vi "SpreadsheetFGV2_Improvements.vi"(0 "Student ID":i32, 1 "FGV Control":T1, 11 "Error In":errorcluster) -> (3 "Time Stamp Out":timestamp, 4 "Message":string, 6 "Names":string[](array[string]), 8 "Output 2D Data":string[][](array[string]), 10 "Checked In?":bool, 12 "Cat Points":i32, 14 "Elapsed Time":dbl, 15 "Error Out":errorcluster)   [LabVIEW 2013]
uses:
  Controls/CSVFGVStates.ctl
  Controls/SpreadsheetColumns.ctl
  <vilib>/Utility/file.llb/Write To Spreadsheet File (string).vi
  <vilib>/Utility/file.llb/Read From Spreadsheet File (string).vi
panel:
  out "Checked In":string
  out "all rows":string[][](array[string])
  in  "Replacement":string
  in  "Student Names":i32(listbox)
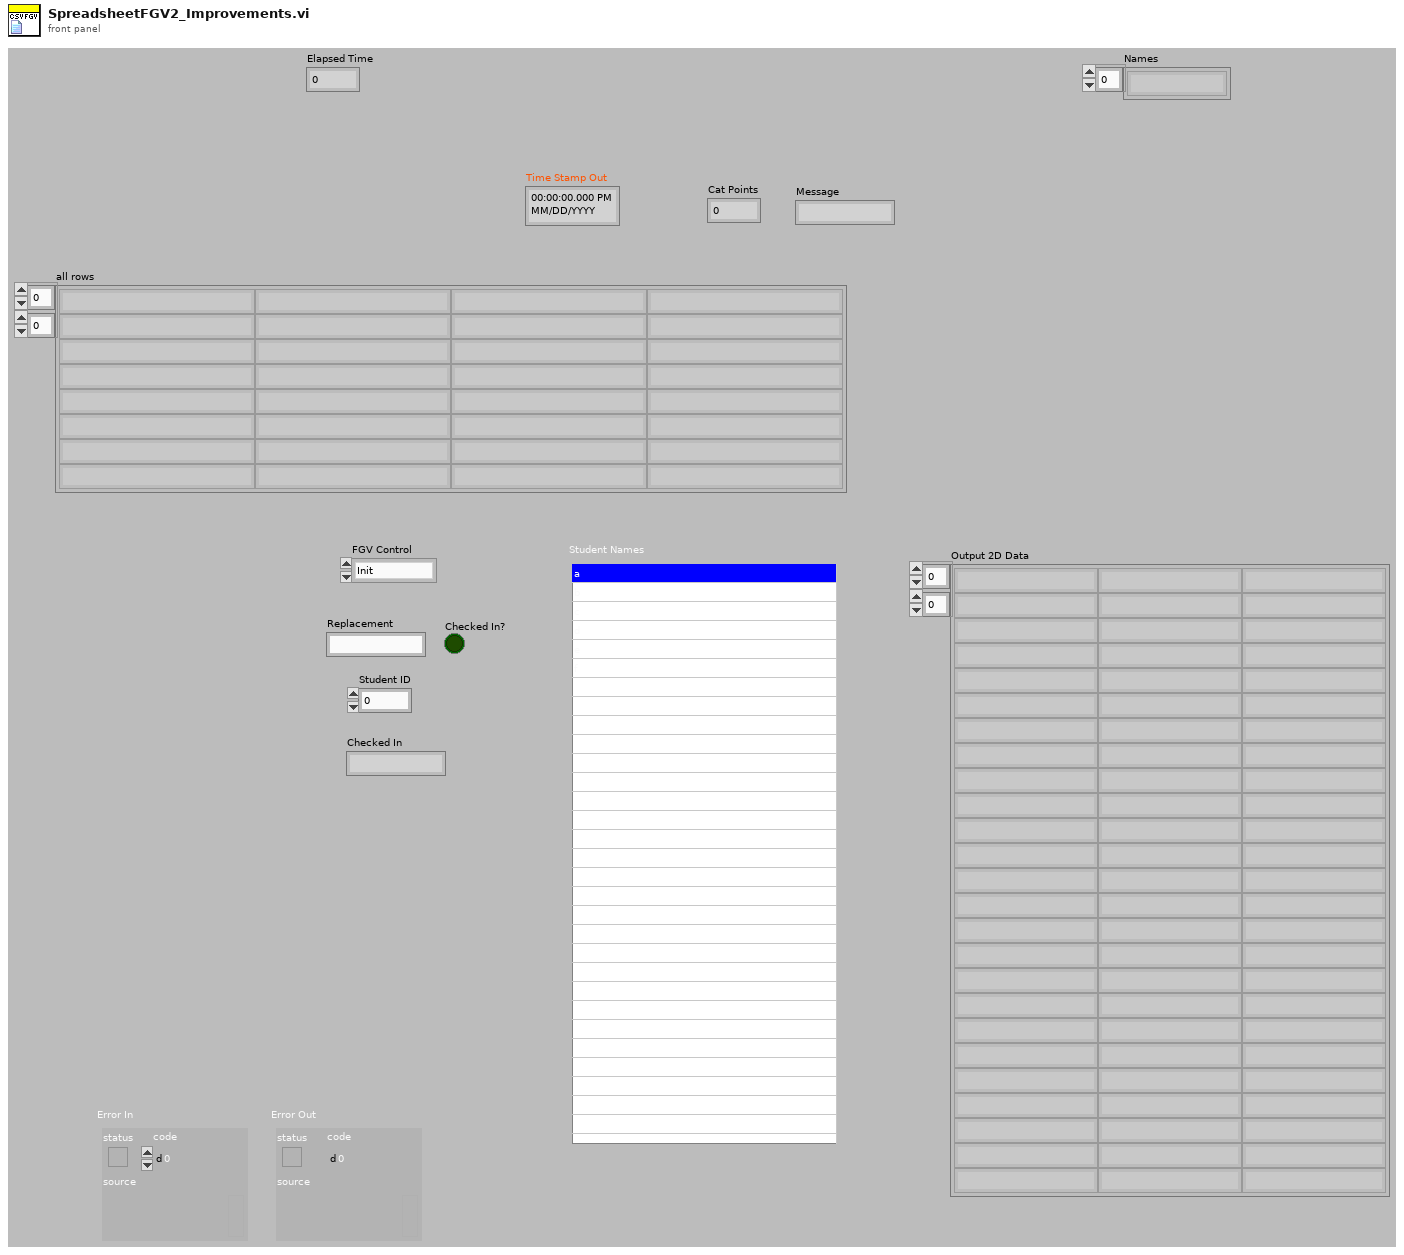
[diagram p1: front panel]
types:
  T1 = typedef "CSVFGVStates.ctl" = enum16{"Init", "Sort", "Check In", "Check Out", "Check Status", "Read CSV", "Close Out"}
  T2 = typedef "SpreadsheetColumns.ctl" = enum16{"Email", "CheckIn", "CheckOut", "Flag", "Hours", "Minutes", "Seconds", "Total Seconds", "Cat Points"}
  T3 = cluster{"Flag":T2, "Check In":T2, "Hours":T2, "Minutes":T2, "Seconds":T2, "Check Out":T2, "Email":T2, "Total Seconds":T2}
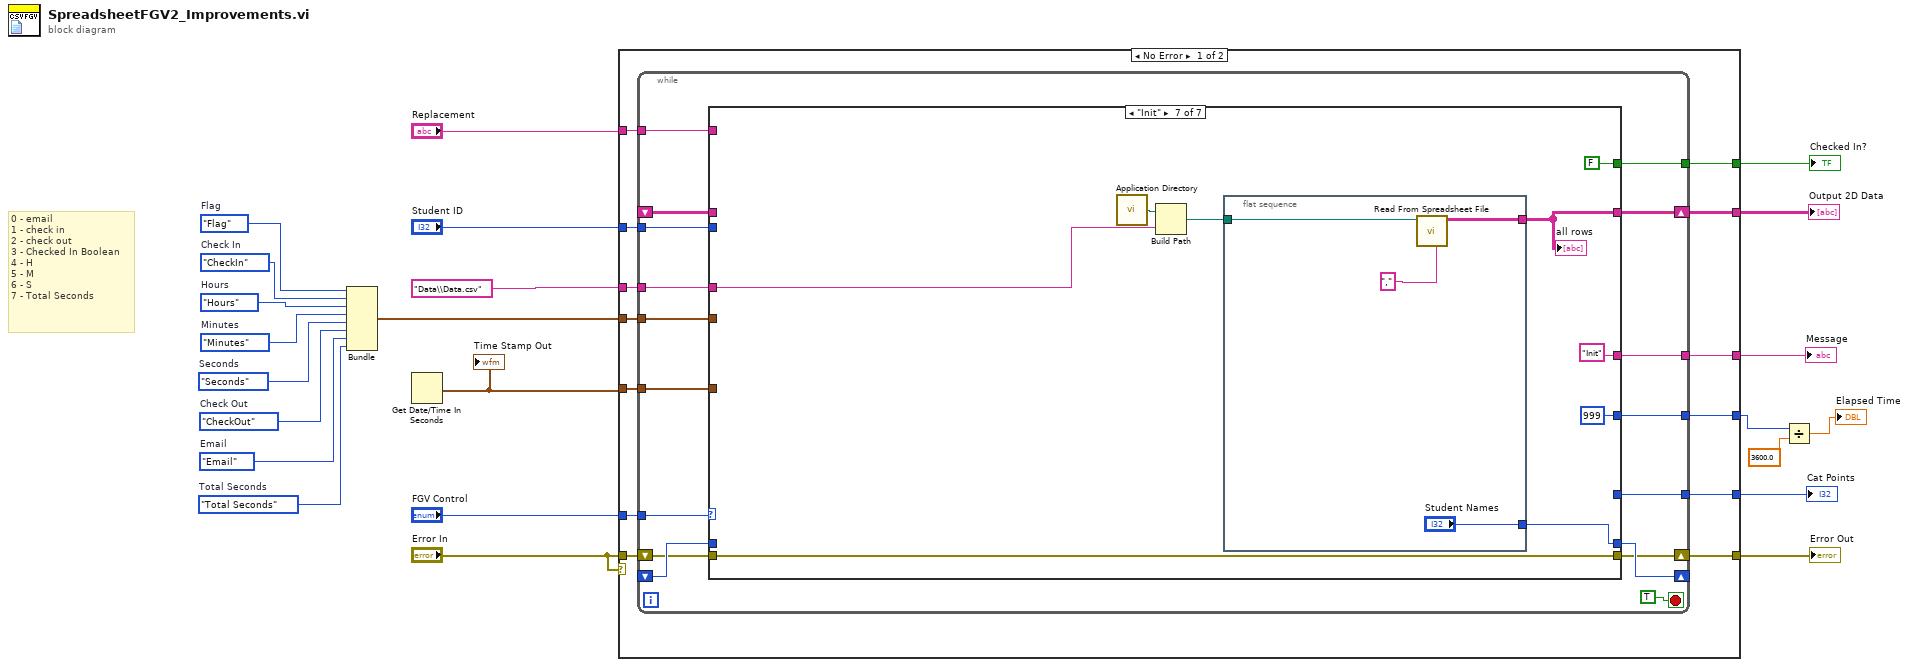
[diagram p0: block diagram]
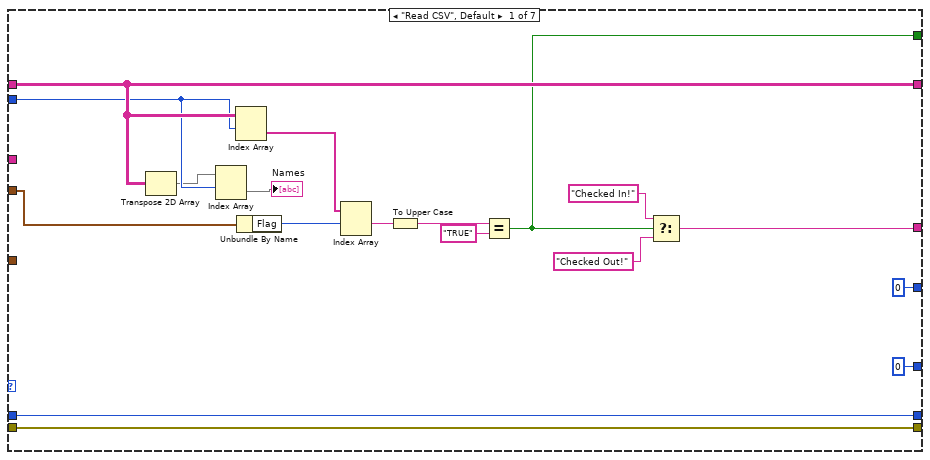
[diagram p2: hidden frame]
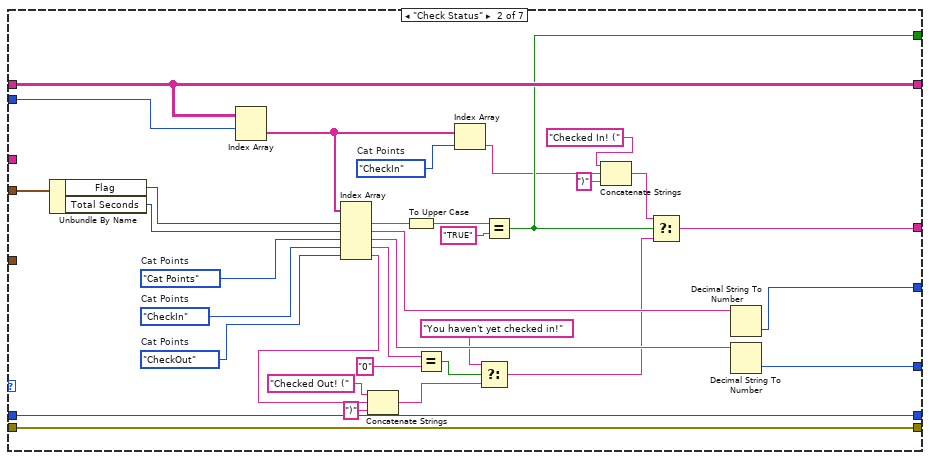
[diagram p3: hidden frame]
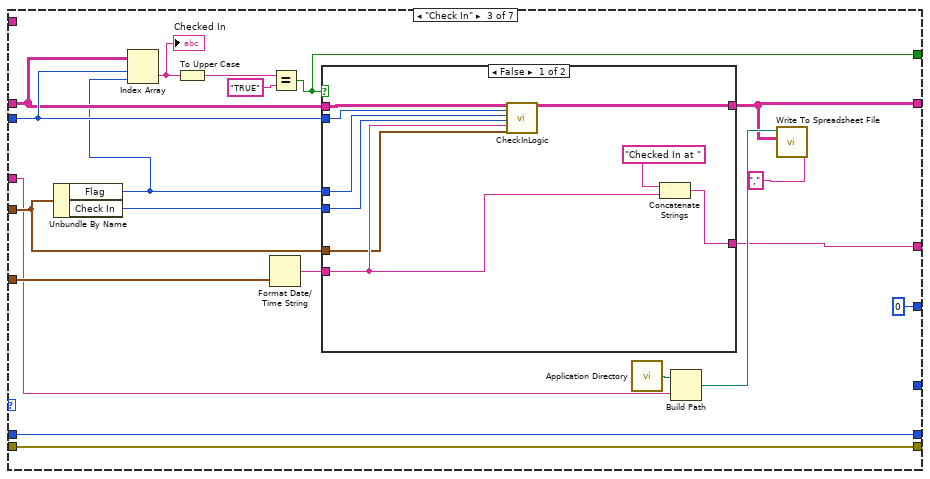
[diagram p4: hidden frame]
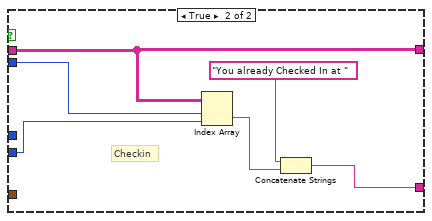
[diagram p5: hidden frame]
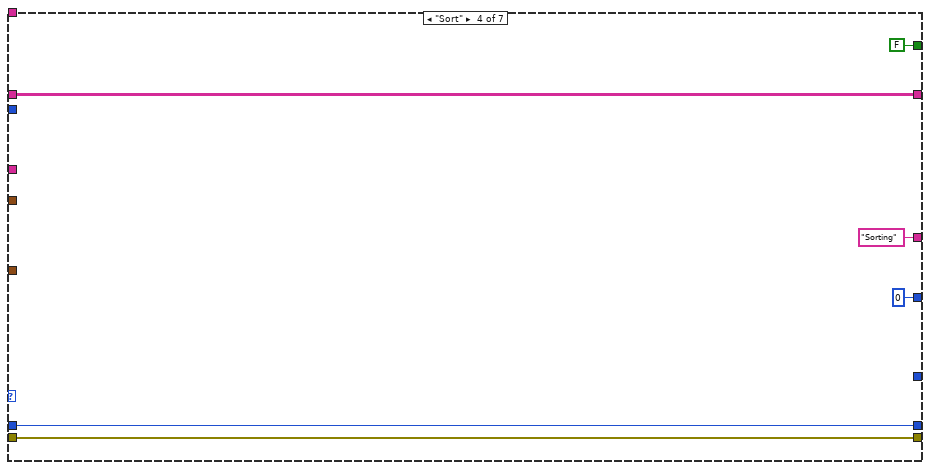
[diagram p6: hidden frame]
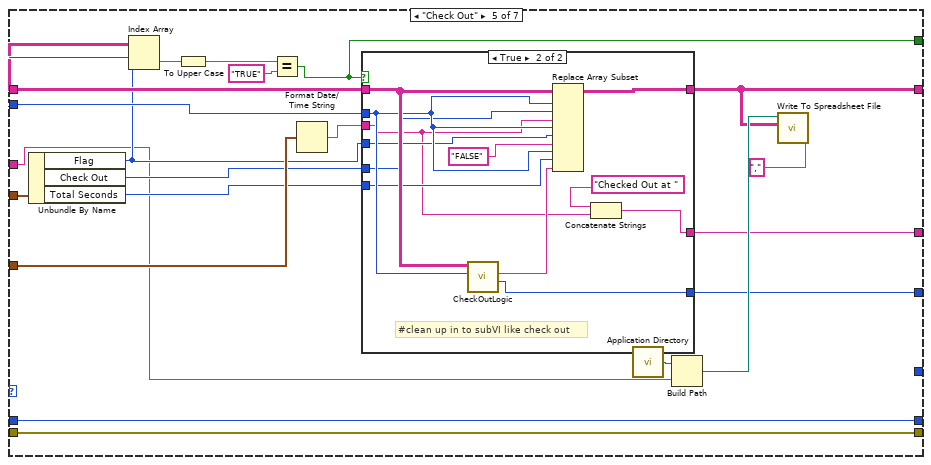
[diagram p7: hidden frame]
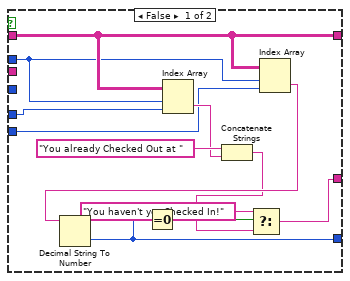
[diagram p8: hidden frame]
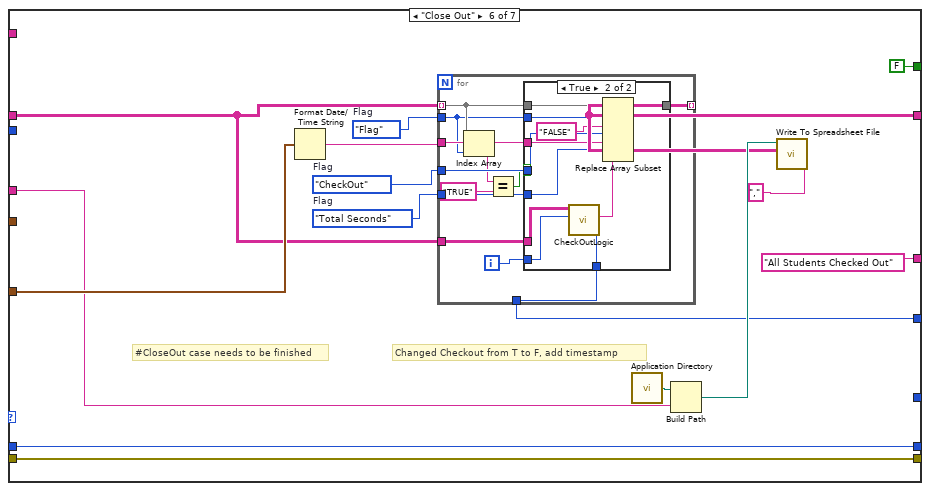
[diagram p9: hidden frame]
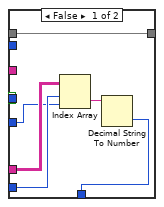
[diagram p10: hidden frame]
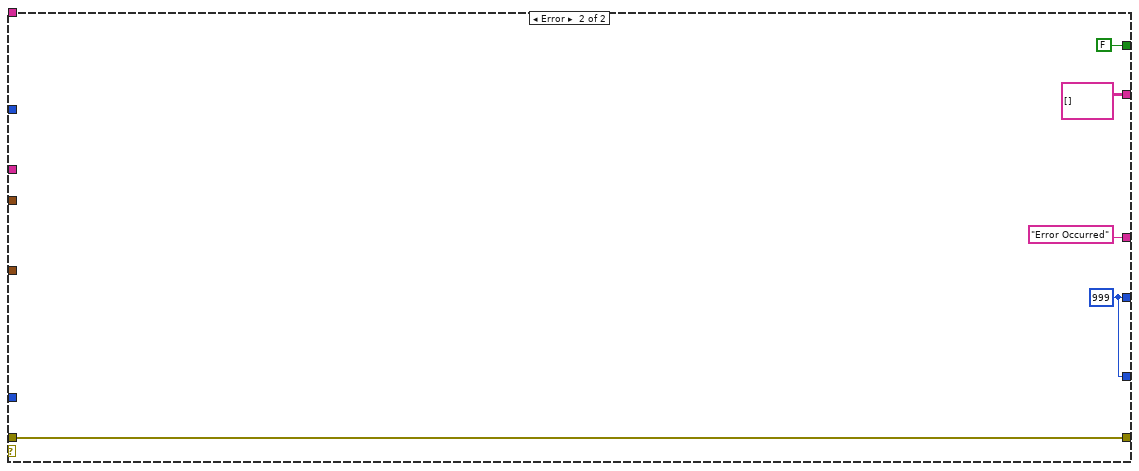
[diagram p11: hidden frame]
diagram:
  w8 = SpreadsheetColumns."Total Seconds"  # Total Seconds
  w9 = SpreadsheetColumns."Email"  # Email
  w10 = SpreadsheetColumns."CheckOut"  # Check Out
  w12 = SpreadsheetColumns."Seconds"  # Seconds
  w13 = SpreadsheetColumns."Minutes"  # Minutes
  w14 = SpreadsheetColumns."Hours"  # Hours
  w16 = SpreadsheetColumns."Flag"  # Flag
  w15 = SpreadsheetColumns."CheckIn"  # Check In
  # "0 - email\n1 - check in\n2 - check out\n3 - Checked In Boolean\n4 - H\n5 - M\n6 - S\n7 - Total Seconds"
  n1 = Bundle("Flag"=w16, "Check In"=w15, "Hours"=w14, "Minutes"=w13, "Seconds"=w12, "Check Out"=w10, "Email"=w9, "Total Seconds"=w8) -> (w11:T3)  [unwired: 1 in]
  n2 = Get Date/Time In Seconds() -> (seconds since 1Jan1904=w5:timestamp)
  "Time Stamp Out" <- w5
  n3 = case shown="No Error" "Error In" {
    tunnel: "FGV Control" -> [w36 _]
    tunnel: "Error In" -> [w34 w254]
    tunnel: [w35 w254] -> w21
    tunnel: "Student ID" -> [w33 _]
    tunnel: w5 -> [w32 _]
    tunnel: "Replacement" -> [w31 _]
    tunnel: [w30 FALSE] -> w7
    tunnel: [w29 string[][] [] ("all rows")] -> w18
    tunnel: [w28 "Error Occurred" ("date/time string")] -> w17
    tunnel: [w27 w250] -> w2
    tunnel: w11 -> [w26 _]
    tunnel: "Data\\Data.csv" ("name or relative path") -> [w25 _]
    tunnel: [w24 w250] -> w4
    frame No Error {
      n4 = while {
        shift-right: [w44] -> w29
        shift-left: _ -> [w39]
        tunnel: w36 -> [w52]
        shift-right: [w51] -> _
        shift-left: _ -> [w50]
        shift-right: [w49] -> w35
        shift-left: w34 -> [w48]
        tunnel: w33 -> [w47]
        tunnel: w32 -> [w46]
        tunnel: w31 -> [w45]
        tunnel: [w43] -> w30
        tunnel: [w42] -> w28
        tunnel: [w41] -> w27
        tunnel: w26 -> [w40]
        tunnel: w25 -> [w38]
        tunnel: [w37] -> w24
        stop <- TRUE stop-if-true
        n5 = case shown="\"Init\"" w52 {
          tunnel: w39 -> [w61 w99 w112 w141 w155 w193 _]
          tunnel: [w70 w104 w122 w145 w164 w204 w244] -> w51
          tunnel: w50 -> [w70 w104 w122 w145 w164 w204 _]
          tunnel: [w71 w105 w124 w146 w166 w206 w243] -> w49
          tunnel: w48 -> [w71 w105 w124 w146 w166 w206 w243]
          tunnel: w47 -> [w60 w95 w113 _ w156 _ _]
          tunnel: w46 -> [_ _ w115 _ w162 w202 _]
          tunnel: w45 -> [_ _ _ _ _ _ _]
          tunnel: [w61 w99 w107 w141 w160 w201 w237] -> w44
          tunnel: [w57 w96 w111 FALSE w149 FALSE FALSE] -> w43
          tunnel: [w62 w100 w116 "Sorting" ("date/time string") w154 "All Students Checked Out" ("date/time string") "Init" ("date/time string")] -> w42
          tunnel: [0 ("Elapsed Seconds") w92 0 ("Elapsed Seconds") 0 ("Elapsed Seconds") w153 w192 999 ("Elapsed Seconds")] -> w41
          tunnel: w40 -> [w56 w98 w110 _ w152 _ _]
          tunnel: w38 -> [_ _ w109 _ w147 w197 w238]
          tunnel: [0 w89 _ _ _ _ _] -> w37
          frame "Read CSV", Default {
            n6 = Transpose 2D Array(2D array=w61) -> (transposed array=w59:string[][])
            n7 = Index Array(array=w59, index (row)=w60) -> (element=→"Names":string[])  [unwired: 1 in]
            n8 = Index Array(array=w61, index (row)=w60) -> (element=w65:string[])  [unwired: 1 in]
            n9 = Unbundle By Name(w56) -> ("Flag"=w55:T2)
            n10 = Index Array(array=w65, index #1=w55) -> (element #1=w68:string)  [unwired: 1 in, 1 out]
            n11 = To Upper Case(1:w68) -> (0:w67:string)
            n12 = Equal?(x=w67, y="TRUE") -> (x = y?=w57:bool)
            n13 = Select(t="Checked In!" ("y"), s=w57, f="Checked Out!" ("y")) -> (s? t:f=w62:string)
          }
          frame "Check Status" {
            w77 = SpreadsheetColumns."CheckIn"  # Cat Points
            w76 = SpreadsheetColumns."CheckOut"  # Cat Points
            w88 = SpreadsheetColumns."CheckIn"  # Cat Points
            w91 = SpreadsheetColumns."Cat Points"  # Cat Points
            n14 = Unbundle By Name(w98) -> ("Flag"=w97:T2, "Total Seconds"=w94:T2)
            n15 = Index Array(array=w99, index (row)=w95) -> (element=w78:string[])  [unwired: 1 in]
            n16 = Index Array(array=w78, index #1=w97, index #2=w94, index #3=w91, index #4=w88, index #5=w76) -> (element #1=w103:string, element #2=w93:string, element #3=w90:string, element #4=w87:string, element #5=w80:string)
            n17 = Concatenate Strings("Checked Out! (" ("y"), w80, ")" ("string")) -> (w81:string)
            n18 = To Upper Case(1:w103) -> (0:w102:string)
            n19 = Equal?(x=w87, y="0") -> (x = y?=w85:bool)
            n20 = Index Array(array=w78, index=w77) -> (element=w74:string)
            n21 = Select(t="You haven't yet checked in!", s=w85, f=w81) -> (s? t:f=w84:string)
            n22 = Equal?(x=w102, y="TRUE") -> (x = y?=w96:bool)
            n23 = Concatenate Strings("Checked In! (" ("y"), w74, ")" ("string")) -> (w72:string)
            n24 = Select(t=w72, s=w96, f=w84) -> (s? t:f=w100:string)
            n25 = Decimal String To Number(string=w93) -> (number=w92:i32)  [unwired: 2 in, 1 out]
            n26 = Decimal String To Number(string=w90) -> (number=w89:i32)  [unwired: 2 in, 1 out]
          }
          frame "Check In" {
            n27 = Unbundle By Name(w110) -> ("Flag"=w108:T2, "Check In"=w114:T2)
            n28 = Index Array(array=w112, index (row)=w113, index (col)=w108) -> (element=w119:string)
            "Checked In" <- w119
            n29 = To Upper Case(1:w119) -> (0:w118:string)
            n30 = Format Date/Time String(seconds (now)=w115) -> (date/time string=w120:string)  [unwired: 2 in]
            n31 = Equal?(x=w118, y="TRUE") -> (x = y?=w111:bool)
            n32 = case shown="False" w111 {
              tunnel: w120 -> [w127 _]
              tunnel: [w131 w140] -> w107
              tunnel: w113 -> [w130 w139]
              tunnel: w112 -> [w132 w140]
              tunnel: [w133 w136] -> w116
              tunnel: w108 -> [w129 _]
              tunnel: w114 -> [w128 w135]
              tunnel: w110 -> [w126 _]
              frame False {
                n33 = call "CheckInLogic.vi"("all rows in"=w132, "Student ID"=w130, "Flag"=w129, "Check In"=w128, "date/time string"=w127, "Time Cluster"=w126) -> ("all rows out"=w131:string[][])  [unwired: 13 in]
                n34 = Concatenate Strings("Checked In at " ("String"), w127) -> (w133:string)
              }
              frame True {
                # "Checkin"
                n35 = Index Array(array=w140, index (row)=w139, index (col)=w135) -> (element=w137:string)
                n36 = Concatenate Strings("You already Checked In at " ("delimiter (\\t)"), w137) -> (w136:string)
              }
            }
            n37 = call <vilib>:"Application Directory.vi"() -> ("Application Directory"=w125:path)
            n38 = Build Path(base path=w125, name or relative path=w109) -> (appended path=w123:path)
            n39 = call-poly <vilib>:"Write To Spreadsheet File.vi"("delimiter (\\t)"="," ("delimiter (\\t)"), "2D data"=w107, "file path (dialog if empty)"=w123) -> ()  [unwired: 5 in, 1 out]
          }
          frame "Sort" {
          }
          frame "Check Out" {
            n40 = Unbundle By Name(w152) -> ("Flag"=w148:T2, "Check Out"=w150:T2, "Total Seconds"=w151:T2)
            n41 = Index Array(array=w155, index (row)=w156, index (col)=w148) -> (element=w159:string)
            n42 = To Upper Case(1:w159) -> (0:w158:string)
            n43 = Equal?(x=w158, y="TRUE") -> (x = y?=w149:bool)
            n44 = Format Date/Time String(seconds (now)=w162) -> (date/time string=w161:string)  [unwired: 2 in]
            n45 = case shown="True" w149 {
              tunnel: w161 -> [_ w180]
              tunnel: [w176 w191] -> w160
              tunnel: w156 -> [w175 w187]
              tunnel: w155 -> [w176 w188]
              tunnel: [w169 w190] -> w154
              tunnel: [w172 w186] -> w153
              tunnel: w151 -> [w174 w185]
              tunnel: w150 -> [w177 w181]
              tunnel: w148 -> [_ w182]
              frame False {
                n46 = Index Array(array=w176, index (row)=w175, index (col)=w177) -> (element=w178:string)
                n47 = Concatenate Strings("You already Checked Out at " ("string"), w178) -> (w170:string)
                n48 = Index Array(array=w176, index (row)=w175, index (col)=w174) -> (element=w173:string)
                n49 = Decimal String To Number(string=w173) -> (number=w172:i32)  [unwired: 2 in, 1 out]
                n50 = Equal To 0?(x=w172) -> (x = 0?=w171:bool)
                n51 = Select(t="You haven't yet Checked In!", s=w171, f=w170) -> (s? t:f=w169:string)
              }
              frame True {
                # "#clean up in to subVI like check out"
                n52 = call "CheckOutLogic.vi"("Student ID"=w187, "all rows"=w188) -> ("Total Elapsed Time"=w186:i32, "Total Seconds Out"=w184:string)  [unwired: 7 in, 1 out]
                n53 = Replace Array Subset(array=w188, new element #1=w180, index (row) #1=w187, index (col) #1=w181, new element #2="FALSE" ("new element/subarray"), index (row) #2=w187, index (col) #2=w182, new element #3=w184, index (row) #3=w187, index (col) #3=w185) -> (w191:string[][])
                n54 = Concatenate Strings("Checked Out at " ("string"), w180) -> (w190:string)
              }
            }
            n55 = call <vilib>:"Application Directory.vi"() -> ("Application Directory"=w167:path)
            n56 = Build Path(base path=w167, name or relative path=w147) -> (appended path=w165:path)
            n57 = call-poly <vilib>:"Write To Spreadsheet File.vi"("delimiter (\\t)"="," ("delimiter (\\t)"), "2D data"=w160, "file path (dialog if empty)"=w165) -> ()  [unwired: 5 in, 1 out]
          }
          frame "Close Out" {
            w194 = SpreadsheetColumns."Total Seconds"  # Flag
            w195 = SpreadsheetColumns."CheckOut"  # Flag
            w196 = SpreadsheetColumns."Flag"  # Flag
            # "#CloseOut case needs to be finished"
            # "Changed Checkout from T to F, add timestamp"
            n58 = Format Date/Time String(seconds (now)=w202) -> (date/time string=w199:string)  [unwired: 2 in]
            n59 = for {
              tunnel: [w219] -> w201 mode=indexing
              tunnel: w193 -> [w212] mode=indexing
              tunnel: w199 -> [w218]
              tunnel: w196 -> [w211]
              tunnel: w195 -> [w217]
              tunnel: w194 -> [w215]
              tunnel: w193 -> [w214]
              tunnel: [w213] -> w192
              i -> [w216]
              n60 = Index Array(array=w212, index=w211) -> (element=w210:string)
              n61 = Equal?(x=w210, y="TRUE") -> (x = y?=w208:bool)
              n62 = case shown="True" w208 {
                tunnel: [w225 w236] -> w219
                tunnel: w218 -> [_ w234]
                tunnel: w217 -> [_ w233]
                tunnel: w216 -> [w223 w232]
                tunnel: w215 -> [w222 w230]
                tunnel: w214 -> [w224 w229]
                tunnel: [w220 w228] -> w213
                tunnel: w212 -> [w225 w227]
                tunnel: w211 -> [_ w226]
                frame False {
                  n63 = Index Array(array=w224, index (row)=w223, index (col)=w222) -> (element=w221:string)
                  n64 = Decimal String To Number(string=w221) -> (number=w220:i32)  [unwired: 2 in, 1 out]
                }
                frame True {
                  n65 = call "CheckOutLogic.vi"("Student ID"=w232, "all rows"=w229) -> ("Total Elapsed Time"=w228:i32, "Total Seconds Out"=w231:string)  [unwired: 7 in, 1 out]
                  n66 = Replace Array Subset(array=w227, new element #1="FALSE" ("new element/subarray"), index #1=w226, new element #2=w234, index #2=w233, new element #3=w231, index #3=w230) -> (w236:string[])
                }
              }
            }
            n67 = call <vilib>:"Application Directory.vi"() -> ("Application Directory"=w207:path)
            n68 = Build Path(base path=w207, name or relative path=w197) -> (appended path=w205:path)
            n69 = call-poly <vilib>:"Write To Spreadsheet File.vi"("delimiter (\\t)"="," ("delimiter (\\t)"), "2D data"=w201, "file path (dialog if empty)"=w205) -> ()  [unwired: 5 in, 1 out]
          }
          frame "Init" {
            n70 = call <vilib>:"Application Directory.vi"() -> ("Application Directory"=w245:path)
            n71 = Build Path(base path=w245, name or relative path=w238) -> (appended path=w242:path)
            n72 = flat-sequence {
              tunnel: w242 -> [w249]
              tunnel: [w248] -> w237
              tunnel: ["Student Names"] -> w244
              frame #0 {
                n73 = call-poly <vilib>:"Read From Spreadsheet File.vi"("delimiter (\\t)"="," ("delimiter (\\t)"), "file path (dialog if empty)"=w249) -> ("all rows"=w248:string[][])  [unwired: 5 in, 4 out]
              }
            }
            "all rows" <- w237
          }
        }
      }
    }
    frame Error {
      w250 = 999 ("Elapsed Seconds")
    }
  }
  "Error Out" <- w21
  "Checked In?" <- w7
  "Output 2D Data" <- w18
  "Message" <- w17
  "Cat Points" <- w4
  n74 = Divide(x=w2, y=3600.0) -> (x/y=→"Elapsed Time":dbl)
